vi "Pre Launch Init.vi"(11 "Timed Loop Controller in":refnum<class "Timed Loop Actor.lvclass">) -> (0 "error out":errorcluster, 3 "Timed Loop Controller out":refnum<class "Timed Loop Actor.lvclass">)   [LabVIEW 2025, in "Timed Loop Actor.lvlib" / "Timed Loop Actor.lvclass"]
uses:
  Timed Loop Actor.lvclass
  Timed Loop Actor.lvclass/Timed Loop Actor.ctl
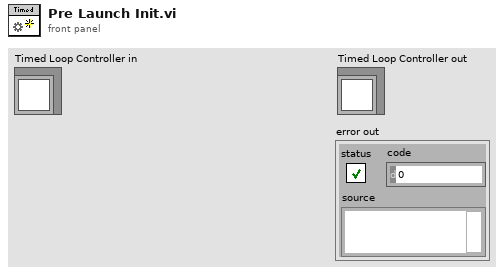
[diagram p1: front panel]
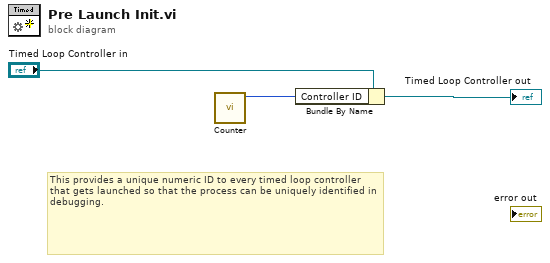
[diagram p0: block diagram]
diagram:
  # "This provides a unique numeric ID to every timed loop controller that gets launched so that the process can be uniquely identified in debugging."
  n1 = call "Counter.vi"() -> ("Numeric"=w1:u32)  [unwired: 11 in]
  n2 = Bundle By Name(cluster="Timed Loop Controller in", "Controller ID"=w1) -> (→"Timed Loop Controller out":refnum<class "Timed Loop Actor.lvclass">)
